vi "Buffered Read, Auto Save.vi"() -> ()   [LabVIEW 2010]
uses:
  <vilib>/measure/matone.llb/Extract Single Tone Information 1 Chan.vi
  <vilib>/Utility/file.llb/Write To Spreadsheet File (I64).vi
  <vilib>/measure/NI_MAPro.lvlib
panel:
  out "XY Graph":cluster{dbl[], dbl[]}(graph)
  out "appended path":path
  out "File Name":string
  in  "save folder":string="Data"
  in  "data file extension":string=".dat"
  in  "time format string (%c)":string="%Y-%m-%d %H-%M.%S"
  in  "Auto Save":bool
  out "Waveform Graph 2":u16[](graph)
  out "ErrCode":i32
  out "ErrMsg":string
  out "Waveform Graph":u16[](graph)
  in  "Range":i32(ring)=2 items=["Not Programmable"=0, "+- 20 V"=27, "+- 10 V"=1, "+- 5 V"=2, "+- 4 V"=28, "+- 2.5 V"=3, "+- 2 V"=29, "+- 1.67 V"=4, "+- 1.25 V"=5, "+- 1 V"=6, "+- .625 V"=7, "+- .5 V"=8, "+- .25 V"=30, "+- .2 V"=31, "+- .1 V"=9, "+- .05 V"=10, "+- .01 V"=11, "+- .005 V"=12, "0 - 10 V"=13, "0 - 5 V"=14, "0 - 4 V"=36, "0 - 2.5 V"=15, "0 - 2 V"=16, "0 - 1.67 V"=17, "0 - 1.25 V"=18, "0 - 1 V"=19, "0 - .5 V"=32, "0 - .25 V"=33, "0 - .2 V"=34, "0 - .1 V"=20, "0 - .02 V"=35, "0 - .01 V"=21, "4 - 20 mA"=22, "2 - 10 mA"=23, "1 - 5 mA"=24, ".5 - 2.5 mA"=25, "0 - 20 mA"=26]
  in  "Rate \n(in samples per second)\n(max rate 8000)":i32=100
  in  "Count\n(high count decreases \nsampling rate)":i32=100
  in  "Board Number":u32
  in  "Channel":i32
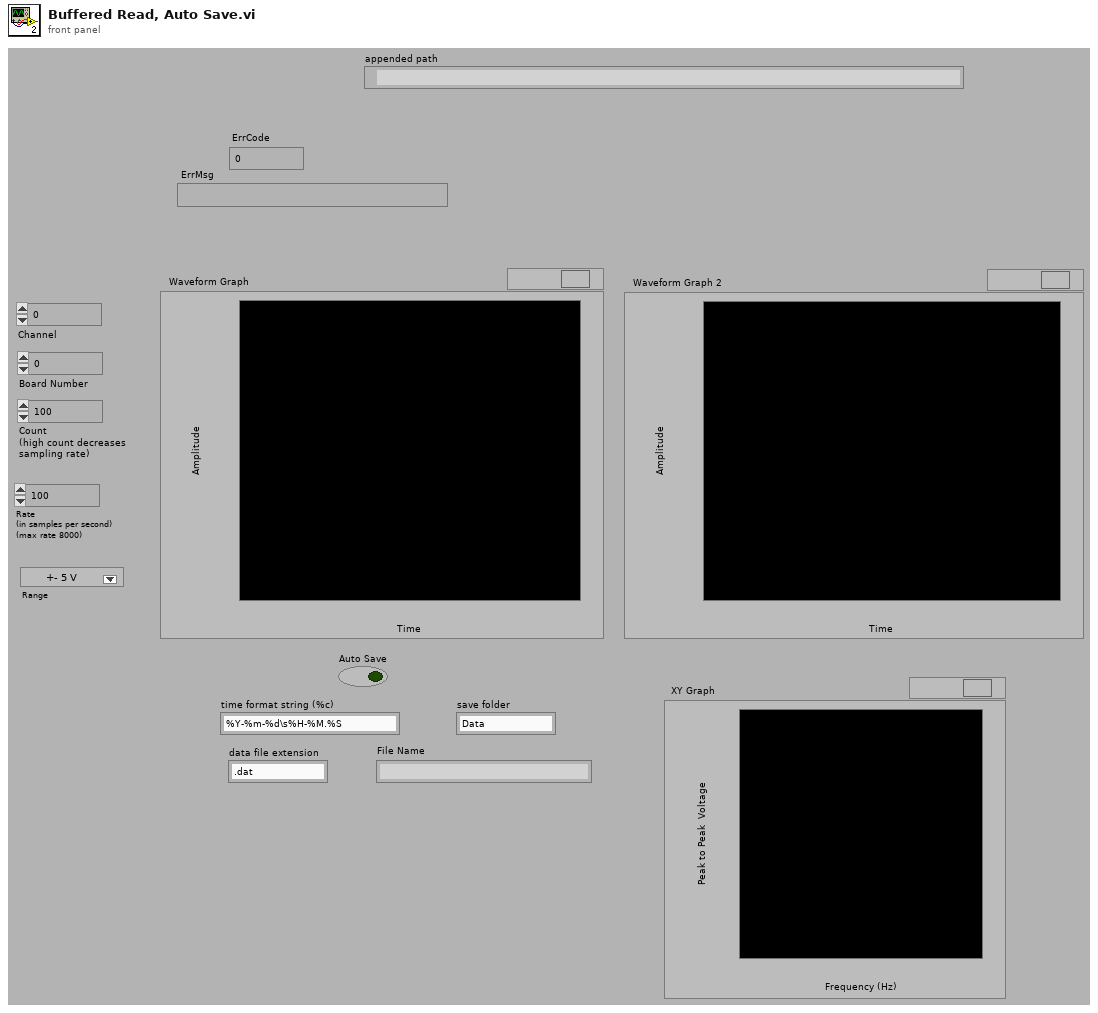
[diagram p1: front panel]
types:
  T1 = typedef "imagedata.ctl" = cluster{"image type":i32, "image depth":i32, "image":u8[], "mask":u8[], "colors":u32[], "Rectangle":cluster{"left":i16, "top":i16, "right":i16, "bottom":i16}}
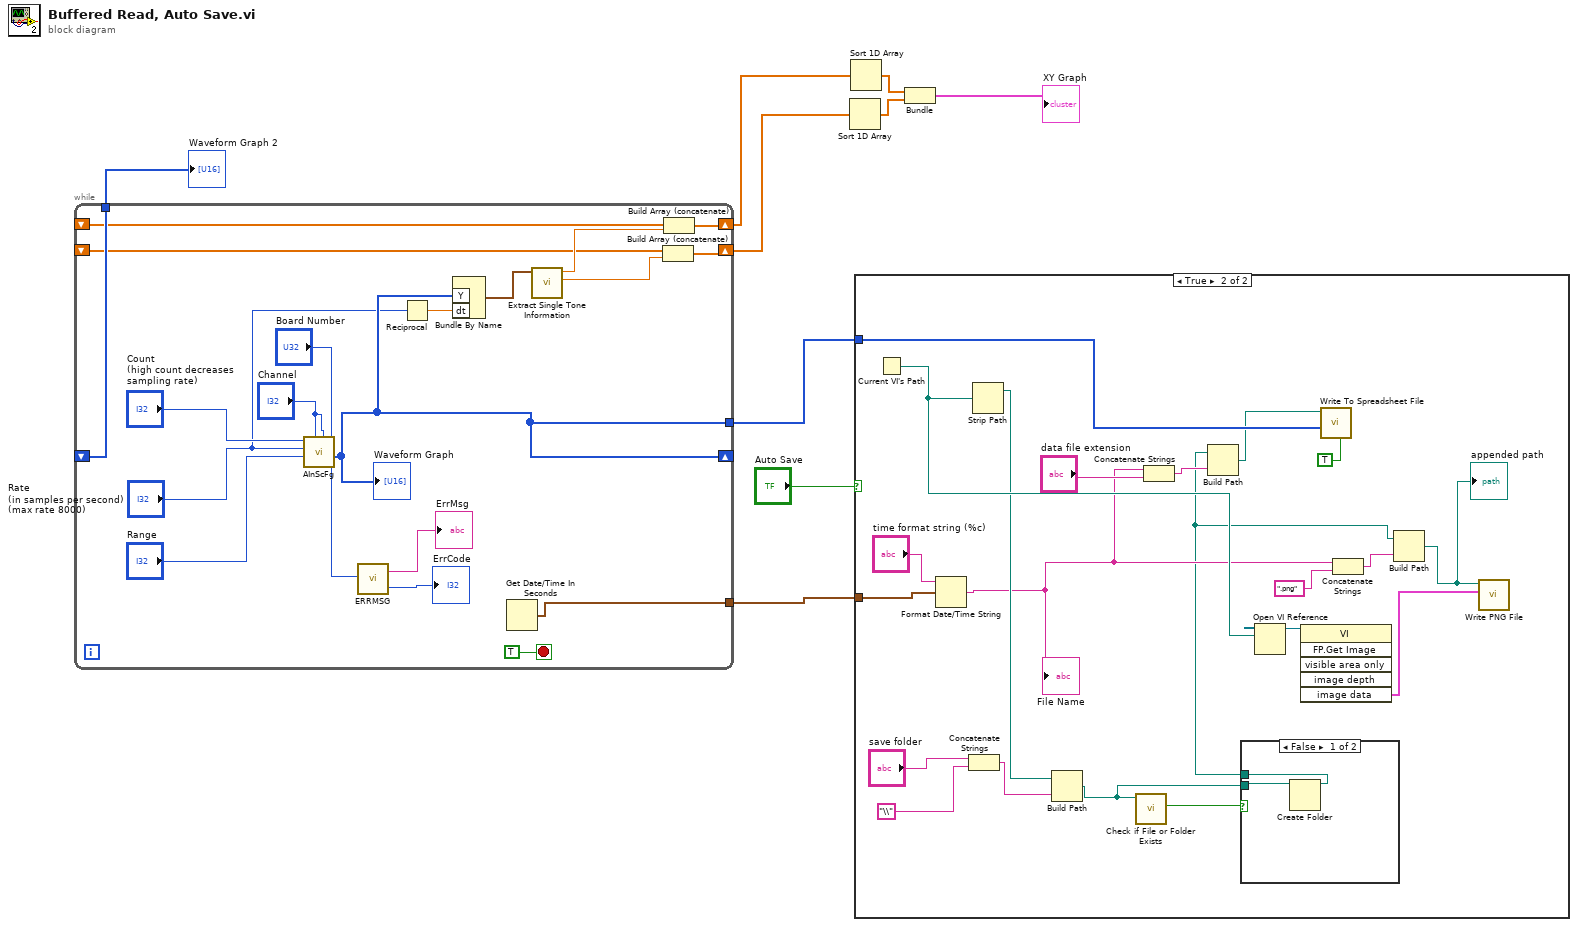
[diagram p0: block diagram]
diagram:
  n1 = while {
    shift-right: [w19] -> _
    shift-left: _ -> [w21]
    tunnel: [w21] -> w9
    tunnel: [w19] -> w7
    tunnel: [w20] -> w6
    shift-right: [w14] -> w2
    shift-left: _ -> [w11]
    shift-right: [w15] -> w1
    shift-left: _ -> [w10]
    stop <- TRUE stop-if-true
    n2 = call <menus>:"AInScFg.VI"("BoardNum"="Board Number", "LowChan"="Channel", "HighChan"="Channel", "Range"="Range", "Rate"="Rate \n(in samples per second)\n(max rate 8000)", "Count"="Count\n(high count decreases \nsampling rate)") -> ("ErrCode"=w25:i32, "ADData"=w19:u16[])  [unwired: 2 in, 1 out]
    "Waveform Graph" <- w19
    n3 = call <menus>:"ERRMSG.VI"("ErrCode"=w25) -> ("ErrMsg"=→"ErrMsg":string, "ErrCode (Out)"=→"ErrCode":i32)
    n4 = Reciprocal(x="Rate \n(in samples per second)\n(max rate 8000)") -> (1/x=w18:dbl)
    n5 = Bundle By Name("Y"=w19, "dt"=w18) -> (w16:waveform(u16))  [unwired: 1 in]
    n6 = Get Date/Time In Seconds() -> (seconds since 1Jan1904=w20:timestamp)
    n7 = call-poly <vilib>:"Extract Single Tone Information.vi"("time signal in"=w16) -> ("detected amplitude"=w12:dbl, "detected frequency"=w13:dbl)  [unwired: 5 in, 4 out]
    n8 = Build Array (concatenate)(w10, w12) -> (w15:dbl[])
    n9 = Build Array (concatenate)(w11, w13) -> (w14:dbl[])
  }
  "Waveform Graph 2" <- w9
  n10 = Sort 1D Array(array=w1) -> (sorted array=w4:dbl[])
  n11 = Sort 1D Array(array=w2) -> (sorted array=w3:dbl[])
  n12 = case shown="True" "Auto Save" {
    tunnel: w7 -> [_ w50]
    tunnel: w6 -> [_ w47]
    frame False {
    }
    frame True {
      n13 = Current VI's Path() -> (path=w44:path)
      n14 = Format Date/Time String(time format string (%c)="time format string (%c)", seconds (now)=w47) -> (date/time string=w32:string)  [unwired: 1 in]
      "File Name" <- w32
      n15 = Concatenate Strings("save folder", "\\") -> (w34:string)
      n16 = Strip Path(path=w44) -> (stripped path=w33:path)  [unwired: 1 out]
      n17 = Build Path(base path=w33, name or relative path=w34) -> (appended path=w35:path)
      n18 = call <vilib>:"Check if File or Folder Exists.vi"("path"=w35) -> ("file or folder exists?"=w31:bool)  [unwired: 8 in, 2 out]
      n19 = Concatenate Strings(w32, "data file extension") -> (w43:string)
      n20 = case shown="False" w31 {
        tunnel: w35 -> [w52 w53]
        tunnel: [w51 w53] -> w30
        frame False {
          n21 = Create Folder(path (use dialog)=w52) -> (created path=w51:path)  [unwired: 2 in, 2 out]
        }
        frame True {
        }
      }
      n22 = Build Path(base path=w30, name or relative path=w43) -> (appended path=w37:path)
      n23 = Open VI Reference(vi path=w44) -> (vi reference=w40:refnum<vi>)  [unwired: 5 in, 1 out]
      n24 = invoke class="VI" method="FP.Get Image"(reference=w40) -> ("image data"=w39:T1)  [unwired: 5 in, 5 out]
      n25 = call-poly <vilib>:"Write To Spreadsheet File.vi"("transpose? (no:F)"=TRUE, "1D data"=w50, "file path (dialog if empty)"=w37) -> ()  [unwired: 5 in, 1 out]
      n26 = Concatenate Strings(w32, ".png") -> (w38:string)
      n27 = Build Path(base path=w30, name or relative path=w38) -> (appended path=w36:path)
      "appended path" <- w36
      n28 = call <vilib>:"Write PNG File.vi"("image data"=w39, "path to PNG file"=w36) -> ()  [unwired: 8 in, 2 out]
    }
  }
  n29 = Bundle(w3, w4) -> (→"XY Graph":cluster{dbl[], dbl[]})  [unwired: 1 in]
